vi "Destroy Window.vi"(8 "error in (no error)":errorcluster, 11 "Window in":refnum<class "Window.lvclass">) -> (0 "error out":errorcluster)   [LabVIEW 2015, in "IBEX Device.lvlib" / "Window.lvclass"]
doc: "Destroys a Window.lvclass object and closes internally managed references."
uses:
  Window.lvclass
  Window.lvclass/Window.ctl
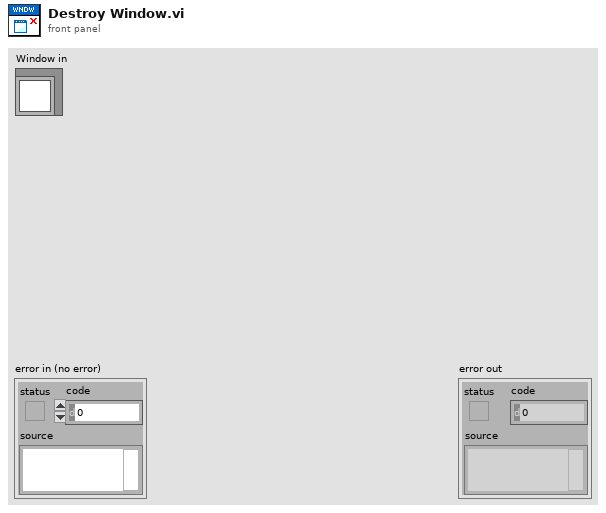
[diagram p1: front panel]
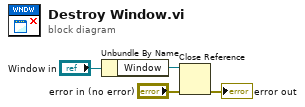
[diagram p0: block diagram]
diagram:
  n1 = Unbundle By Name("Window in") -> ("Window"=w3:refnum<vi>)
  n2 = Close Reference(reference=w3, error in (no error)="error in (no error)") -> (error out=→"error out":errorcluster)
